vi "Initialize Sessions - NSess.vi"(6 "initialize and close session behavior":T1, 7 "serial configuration":T2, 8 "error in":errorcluster, 9 "reset":bool, 11 "session reservation in":refnum<class "Session Reservation.lvclass">) -> (0 "error out":errorcluster, 1 "channel lists":string[](array[string]), 2 "sessions":refnum<visa-resource-name>[](array[refnum]), 3 "session reservation out":refnum<class "Session Reservation.lvclass">)   [LabVIEW 2025, in "Keysight 34461A DMM Instrument.lvlib"]
doc: "Create the 34401 driver sessions from the <b>session reservation in</b>."
uses:
  Keysight 34461A DMM Instrument.lvlib
  <vilib>/Plug-In SDKs/Clients/Session Management V1/Session Reservation/Session Reservation.lvclass
  <vilib>/Plug-In SDKs/Clients/Session Management V1/Session Reservation/Initialize and Close Session Behavior.ctl
  45c620b4-8dfe-4e16-a6c4-07c60f9a1249.vi
  Session Factory/Session Factory.lvclass
  C:/Program Files/National Instruments/LabVIEW 2025/vi.lib/Plug-In SDKs/Sessions/Instrument/ISession Factory/ISession Factory.lvclass
  <vilib>/Plug-In SDKs/Clients/Session Management V1/Session Reservation/Initialize Sessions with Retry.vi
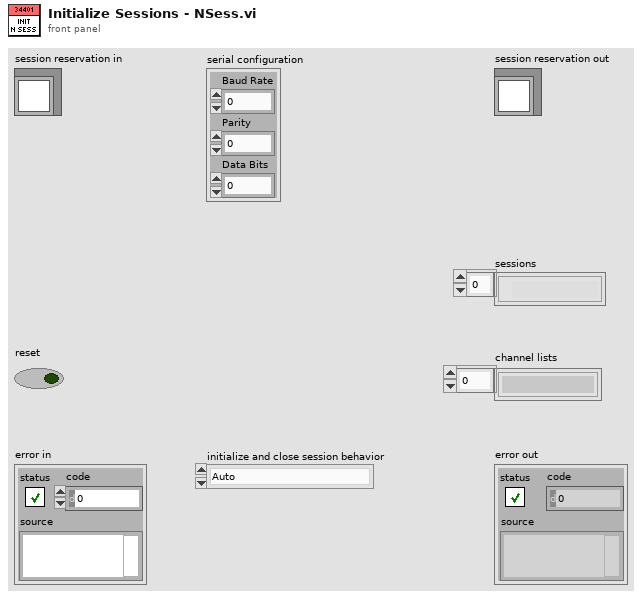
[diagram p1: front panel]
types:
  T1 = typedef "NI Session Management V1 Client.lvlib/Session Reservation.lvclass/Initialize and Close Session Behavior.ctl" = enum16{"Auto", "Initialize and Close", "Attach and Detach", "Initialize and Detach", "Attach and Close"}
  T2 = cluster{"Baud Rate":u32, "Parity":u16, "Data Bits":u16}
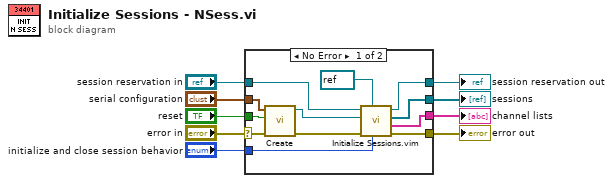
[diagram p0: block diagram]
diagram:
  n1 = case shown="No Error" "error in" {
    selector: "error in" -> [w20 w23]
    tunnel: [w15 w23] -> w8
    tunnel: [w17 w22] -> w6
    tunnel: "session reservation in" -> [w18 w22]
    tunnel: "serial configuration" -> [w21 _]
    tunnel: "reset" -> [w19 _]
    tunnel: [w14 _] -> w2
    tunnel: [w13 _] -> w4
    tunnel: "initialize and close session behavior" -> [w10 _]
    frame No Error {
      n2 = call "Create.vi"("error in"=w20, "reset"=w19, "serial configuration"=w21) -> ("error out"=w16:errorcluster, "session factory out"=w12:refnum<class "Session Factory.lvclass">)  [unwired: 7 in]
      n3 = call "Initialize Sessions.vim"("initialize and close session behavior"=w10, "session type"=refnum<visa-resource-name> refnum ("session"), "error in"=w16, "session factory"=w12, "session reservation in"=w18) -> ("error out"=w15:errorcluster, "channel lists"=w13:string[], "sessions"=w14:refnum<visa-resource-name>[], "session reservation out"=w17:refnum<class "Session Reservation.lvclass">)  [unwired: 3 in]
    }
    frame Error {
    }
  }
  "error out" <- w8
  "session reservation out" <- w6
  "channel lists" <- w4
  "sessions" <- w2
